vi "ZE_Recorder_CreatePath.vi"(8 "date time rec":T1, 10 "File Path Base":path, 11 "File Name":string) -> (2 "time Stamp":string, 3 "file path":path)   [LabVIEW 2025, in "ZE_Recorder.lvlib"]
doc: "ZE_Recorder_CreatePath.vi\n----------------------------------------------\nThe VI creates an unique path for the measurement file using the current timestamp and the defined path base and filename\n\nInputs:\n---------------------\n- date time rec : Cluster; \n- File Path Base : Path; \n- File Name : String; \n\nOutputs:\n---------------------\n- time Stamp : String; \n- file path : Path; \n\n----------------------------------------------\n02.06.2016\nZühlke Engineering AG\nCH-8952 Schlieren\nwww.zuehlke.com\n\nZE_Recorder_CreatePath.vi\n----------------------------------------------\ncreates the unique path for the measurement file\n\nInputs:\n---------------------\n- date time rec : Cluster; \n- File Path Base : Path; \n- File Name : String; \n\nOutputs:\n---------------------\n- file path : Path; \n\n----------------------------------------------\n27.05.2016\nZühlke Engineering AG\nCH-8952 Schlieren\nwww.zuehlke.com"
uses:
  ZE_Recorder.lvlib
  <vilib>/Utility/miscctls.llb/LVDateTimeRec.ctl
panel:
  # "Connector Pane"
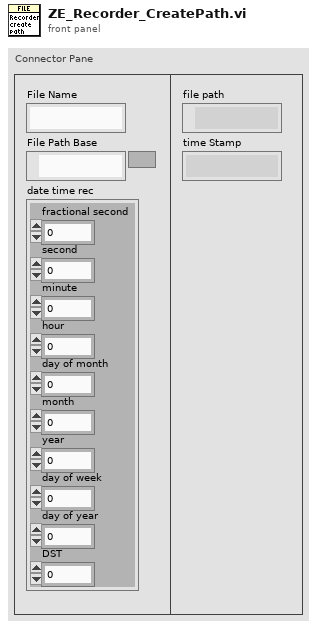
[diagram p1: front panel]
types:
  T1 = typedef "LVDateTimeRec.ctl" = cluster{"fractional second":dbl, "second":i32, "minute":i32, "hour":i32, "day of month":i32, "month":i32, "year":i32, "day of week":i32, "day of year":i32, "DST":i32}
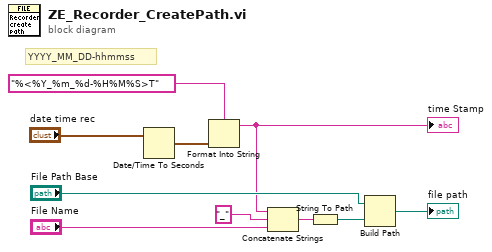
[diagram p0: block diagram]
diagram:
  # "YYYY_MM_DD-hhmmss"
  n1 = Date/Time To Seconds(2:"date time rec") -> (0:w1:timestamp)  [unwired: 1 in]
  n2 = Format Into String(format string="%<%Y_%m_%d-%H%M%S>T", w1) -> (resulting string=w2:string)  [unwired: 2 in, 1 out]
  "time Stamp" <- w2
  n3 = Concatenate Strings(w2, "_", "File Name") -> (w8:string)
  n4 = String To Path(string=w8) -> (path=w6:path)
  n5 = Build Path(base path="File Path Base", name or relative path=w6) -> (appended path=→"file path":path)
